vi "Math-updater-w--for-same-SpVar-names-03022016.vi"(0 "Sp_Id_Arr":string[](array[string]), 1 "Math Expressions":string[](array[string]), 2 "Pr_Id_Arr":string[](array[string]), 3 "LP-Cnt_4_Reac":string[](array[string]), 4 "LP_IDs":string[](array[string])) -> (5 "New Total Pr IDs":string[](array[string]), 6 "Math-w/-ch-VarID":string[](array[string]))   [LabVIEW 2014]
doc: "This VI checks if the variable and species name are same. If they are, then the math is updated with the new variable name in order to distinguish their value."
panel:
  out "j":i32
  out "k":i32
  out "New Pr IDs":string[](array[string])
  out "New LP IDs":string[](array[string])
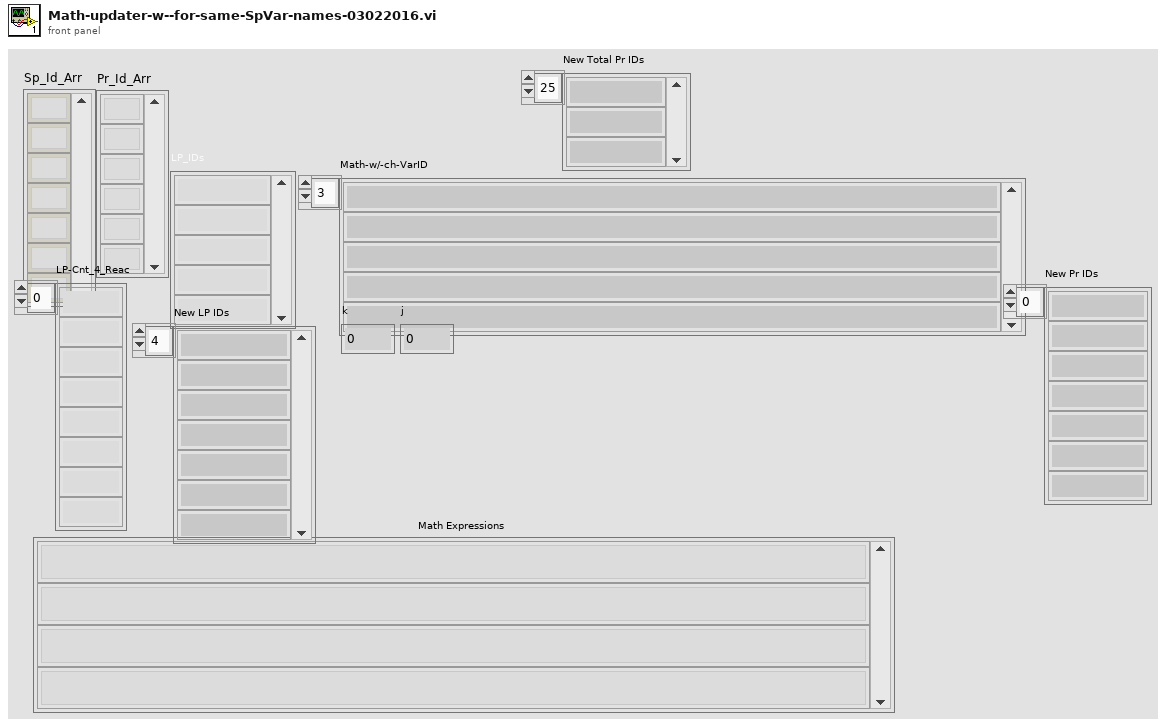
[diagram p1: front panel]
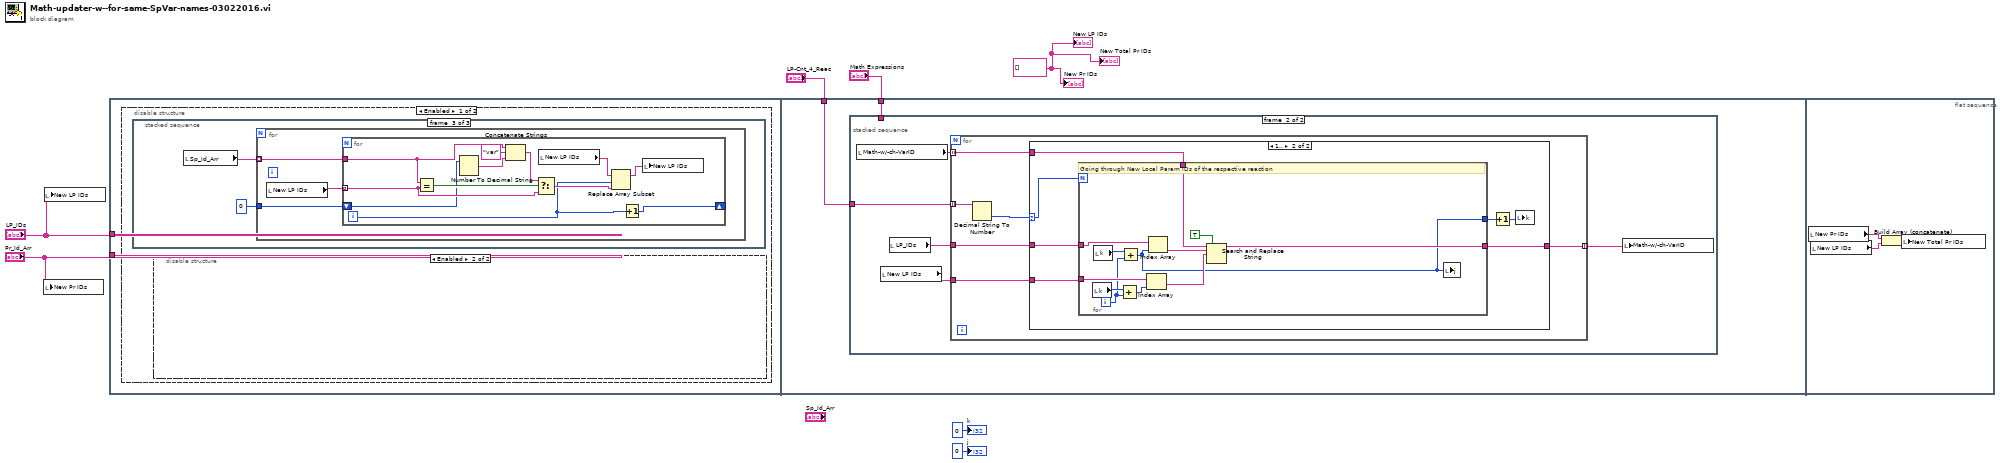
[diagram p0: block diagram]
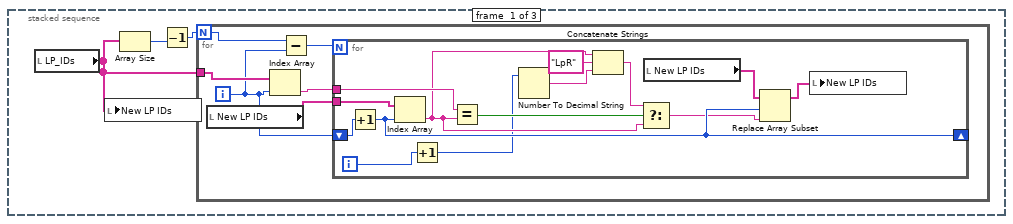
[diagram p2: hidden frame]
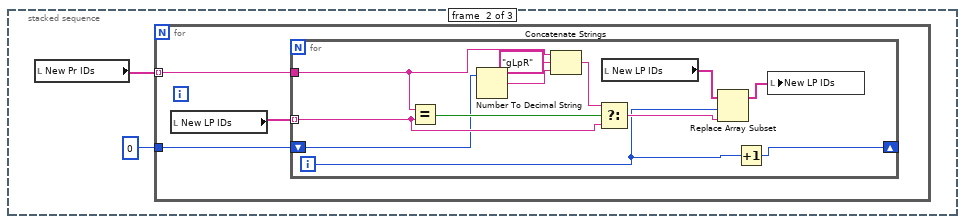
[diagram p3: hidden frame]
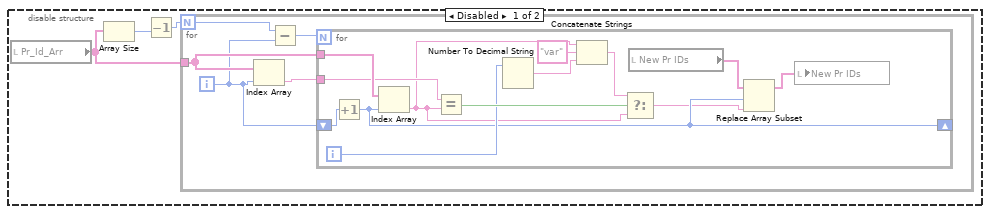
[diagram p4: hidden frame]
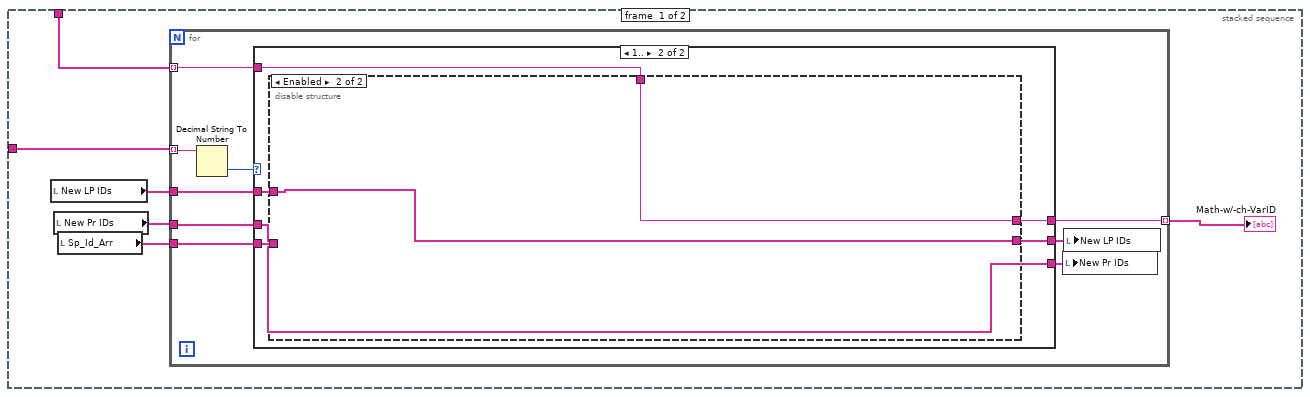
[diagram p6: hidden frame]
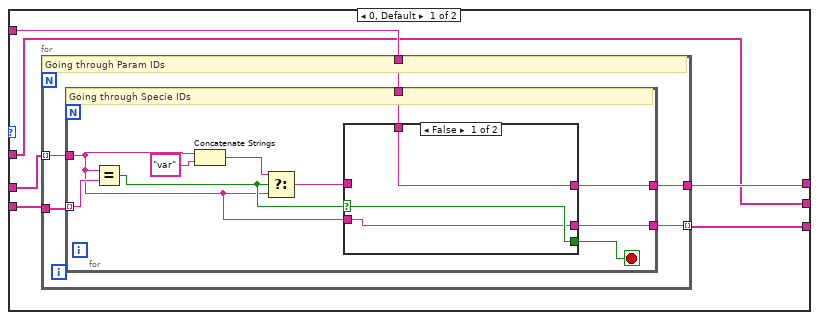
[diagram p7: hidden frame]
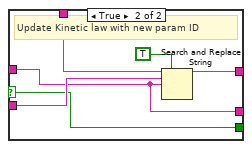
[diagram p8: hidden frame]
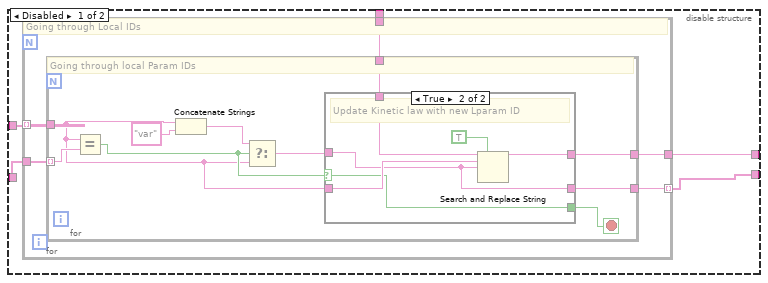
[diagram p9: hidden frame]
diagram:
  w7 = string[] [] ("New LP IDs")
  n1 = local write "New Pr IDs"("Pr_Id_Arr") -> ()
  n2 = local write "New LP IDs"("LP_IDs") -> ()
  n3 = flat-sequence {
    tunnel: "Pr_Id_Arr" -> [_]
    tunnel: "LP_IDs" -> [_]
    tunnel: "Math Expressions" -> [w87]
    tunnel: "LP-Cnt_4_Reac" -> [w86]
    frame #0 {
      n4 = disable-structure shown="Enabled" {
        frame Enabled {
          n5 = stacked-sequence {
            frame #0 {
              n6 = local read "LP_IDs"() -> (w8:string[])
              n7 = local write "New LP IDs"(w8) -> ()
              n8 = Array Size(array=w8) -> (size(s)=w10:i32)
              n9 = Decrement(x=w10) -> (x-1=w9:i32)
              n10 = for {
                N: w9 -> [w16]
                tunnel: w8 -> [w14]
                i -> [w12]
                n11 = local read "New LP IDs"() -> (w11:string[])
                n12 = Index Array(array=w14, index=w12) -> (element=w13:string)
                n13 = Subtract(x=w16, y=w12) -> (x-y=w15:i32)
                n14 = for {
                  N: w15 -> [_]
                  tunnel: w13 -> [w30]
                  shift-right: [w22] -> _
                  shift-left: w12 -> [w28]
                  tunnel: w11 -> [w17]
                  i -> [w19]
                  n15 = Increment(x=w28) -> (x+1=w22:i32)
                  n16 = Index Array(array=w17, index=w22) -> (element=w24:string)
                  n17 = Increment(x=w19) -> (x+1=w18:i32)
                  n18 = Equal?(x=w30, y=w24) -> (x = y?=w29:bool)
                  n19 = Number To Decimal String(number=w18) -> (decimal integer string=w25:string)  [unwired: 1 in]
                  n20 = Concatenate Strings(w24, "LpR" ("string"), w25) -> (w27:string)
                  n21 = Select(t=w27, s=w29, f=w24) -> (s? t:f=w21:string)
                  n22 = local read "New LP IDs"() -> (w23:string[])
                  n23 = Replace Array Subset(array=w23, new element=w21, index=w22) -> (w20:string[])
                  n24 = local write "New LP IDs"(w20) -> ()
                }
              }
            }
            frame #1 {
              n25 = local read "New Pr IDs"() -> (w32:string[])
              n26 = for {
                tunnel: w32 -> [w35] mode=indexing
                tunnel: 0 -> [w33]
                n27 = local read "New LP IDs"() -> (w34:string[])
                n28 = for {
                  tunnel: w35 -> [w40]
                  tunnel: w34 -> [w39] mode=indexing
                  shift-right: [w36] -> _
                  shift-left: w33 -> [w38]
                  i -> [w37]
                  n29 = Equal?(x=w40, y=w39) -> (x = y?=w47:bool)
                  n30 = Number To Decimal String(number=w38) -> (decimal integer string=w44:string)  [unwired: 1 in]
                  n31 = Concatenate Strings(w40, "gLpR" ("string"), w44) -> (w46:string)
                  n32 = Select(t=w46, s=w47, f=w39) -> (s? t:f=w42:string)
                  n33 = local read "New LP IDs"() -> (w43:string[])
                  n34 = Replace Array Subset(array=w43, new element=w42, index=w37) -> (w41:string[])
                  n35 = Increment(x=w37) -> (x+1=w36:i32)
                  n36 = local write "New LP IDs"(w41) -> ()
                }
              }
            }
            frame #2 {
              n37 = local read "Sp_Id_Arr"() -> (w49:string[])
              n38 = for {
                tunnel: w49 -> [w52] mode=indexing
                tunnel: 0 -> [w50]
                n39 = local read "New LP IDs"() -> (w51:string[])
                n40 = for {
                  tunnel: w52 -> [w57]
                  tunnel: w51 -> [w56] mode=indexing
                  shift-right: [w53] -> _
                  shift-left: w50 -> [w55]
                  i -> [w54]
                  n41 = Equal?(x=w57, y=w56) -> (x = y?=w64:bool)
                  n42 = Number To Decimal String(number=w55) -> (decimal integer string=w61:string)  [unwired: 1 in]
                  n43 = Concatenate Strings(w57, "var" ("string"), w61) -> (w63:string)
                  n44 = Select(t=w63, s=w64, f=w56) -> (s? t:f=w59:string)
                  n45 = local read "New LP IDs"() -> (w60:string[])
                  n46 = Replace Array Subset(array=w60, new element=w59, index=w54) -> (w58:string[])
                  n47 = Increment(x=w54) -> (x+1=w53:i32)
                  n48 = local write "New LP IDs"(w58) -> ()
                }
              }
            }
          }
          n49 = disable-structure shown="Enabled" {
            frame Disabled {
              n50 = local read "Pr_Id_Arr"() -> (w65:string[])
              n51 = Array Size(array=w65) -> (size(s)=w66:i32)
              n52 = Decrement(x=w66) -> (x-1=w67:i32)
              n53 = for {
                N: w67 -> [w72]
                tunnel: w65 -> [w70]
                i -> [w68]
                n54 = Index Array(array=w70, index=w68) -> (element=w69:string)
                n55 = Subtract(x=w72, y=w68) -> (x-y=w71:i32)
                n56 = for {
                  N: w71 -> [_]
                  tunnel: w70 -> [w85]
                  tunnel: w69 -> [w84]
                  shift-right: [w75] -> _
                  shift-left: w68 -> [w82]
                  i -> [w78]
                  n57 = Increment(x=w82) -> (x+1=w75:i32)
                  n58 = Index Array(array=w85, index=w75) -> (element=w77:string)
                  n59 = Equal?(x=w84, y=w77) -> (x = y?=w83:bool)
                  n60 = Number To Decimal String(number=w78) -> (decimal integer string=w79:string)  [unwired: 1 in]
                  n61 = Concatenate Strings(w77, "var" ("string"), w79) -> (w81:string)
                  n62 = Select(t=w81, s=w83, f=w77) -> (s? t:f=w74:string)
                  n63 = local read "New Pr IDs"() -> (w76:string[])
                  n64 = Replace Array Subset(array=w76, new element=w74, index=w75) -> (w73:string[])
                  n65 = local write "New Pr IDs"(w73) -> ()
                }
              }
            }
            frame Enabled {
            }
          }
        }
        frame Disabled {
        }
      }
    }
    frame #1 {
      n66 = stacked-sequence {
        tunnel: w87 -> [w93 _]
        tunnel: w86 -> [w92 w174]
        frame #0 {
          n67 = local read "New LP IDs"() -> (w91:string[])
          n68 = local read "New Pr IDs"() -> (w90:string[])
          n69 = local read "Sp_Id_Arr"() -> (w89:string[])
          n70 = for {
            tunnel: w93 -> [w98] mode=indexing
            tunnel: w92 -> [w102] mode=indexing
            tunnel: w91 -> [w100]
            tunnel: w89 -> [w99]
            tunnel: [w97] -> w88 mode=indexing
            tunnel: w90 -> [w96]
            n71 = Decimal String To Number(string=w102) -> (number=w101:i32)  [unwired: 2 in, 1 out]
            n72 = case shown="1.." w101 {
              tunnel: w100 -> [w103 w138]
              tunnel: w99 -> [w106 w137]
              tunnel: w98 -> [w107 w136]
              tunnel: [w108 w135] -> w97
              tunnel: w96 -> [w105 w134]
              tunnel: [w104 w134] -> w95
              tunnel: [w103 w133] -> w94
              frame 0, Default {
                n73 = for {
                  tunnel: w105 -> [w113] mode=indexing
                  tunnel: w106 -> [w112]
                  tunnel: w107 -> [w111]
                  tunnel: [w110] -> w108
                  tunnel: [w109] -> w104 mode=indexing
                  # "Going through Param IDs"
                  n74 = for {
                    tunnel: w113 -> [w117]
                    tunnel: w112 -> [w123] mode=indexing
                    tunnel: w111 -> [w118]
                    tunnel: [w116] -> w110
                    tunnel: [w114] -> w109
                    stop <- w115 stop-if-true
                    # "Going through Specie IDs"
                    n75 = Equal?(x=w117, y=w123) -> (x = y?=w120:bool)
                    n76 = Concatenate Strings(w117, "var") -> (w122:string)
                    n77 = Select(t=w122, s=w120, f=w117) -> (s? t:f=w119:string)
                    n78 = case shown="False" w120 {
                      selector: w120 -> [w125 w128]
                      tunnel: w119 -> [_ w127]
                      tunnel: w118 -> [w126 w131]
                      tunnel: w117 -> [w124 w130]
                      tunnel: [w126 w129] -> w116
                      tunnel: [w125 w128] -> w115
                      tunnel: [w124 w127] -> w114
                      frame False {
                      }
                      frame True {
                        # "Update Kinetic law with new param ID"
                        n79 = Search and Replace String(replace all?=TRUE ("replace all? (F)"), input string=w131, search string=w130, replace string=w127) -> (result string=w129:string)  [unwired: 4 in, 3 out]
                      }
                    }
                  }
                }
              }
              frame 1.. {
                n80 = disable-structure shown="Enabled" {
                  disable-tunnel: w138 -> [w143 w168]
                  disable-tunnel: w137 -> [w142 _]
                  disable-tunnel: w136 -> [w141 w169]
                  disable-tunnel: [w140 w169] -> w135
                  disable-tunnel: [w139 w168] -> w133
                  frame Disabled {
                    n81 = for {
                      tunnel: w143 -> [w148] mode=indexing
                      tunnel: w142 -> [w147]
                      tunnel: w141 -> [w146]
                      tunnel: [w145] -> w140
                      tunnel: [w144] -> w139 mode=indexing
                      # "Going through Local IDs"
                      n82 = for {
                        tunnel: w148 -> [w152]
                        tunnel: w147 -> [w158] mode=indexing
                        tunnel: w146 -> [w153]
                        tunnel: [w151] -> w145
                        tunnel: [w149] -> w144
                        stop <- w150 stop-if-true
                        # "Going through local Param IDs"
                        n83 = Equal?(x=w152, y=w158) -> (x = y?=w155:bool)
                        n84 = Concatenate Strings(w152, "var") -> (w157:string)
                        n85 = Select(t=w157, s=w155, f=w152) -> (s? t:f=w154:string)
                        n86 = case shown="True" w155 {
                          selector: w155 -> [w160 w163]
                          tunnel: w154 -> [_ w162]
                          tunnel: w153 -> [w161 w166]
                          tunnel: w152 -> [w159 w165]
                          tunnel: [w161 w164] -> w151
                          tunnel: [w160 w163] -> w150
                          tunnel: [w159 w162] -> w149
                          frame False {
                          }
                          frame True {
                            # "Update Kinetic law with new Lparam ID"
                            n87 = Search and Replace String(replace all?=TRUE ("replace all? (F)"), input string=w166, search string=w165, replace string=w162) -> (result string=w164:string)  [unwired: 4 in, 3 out]
                          }
                        }
                      }
                    }
                  }
                  frame Enabled {
                  }
                }
              }
            }
            n88 = local write "New Pr IDs"(w95) -> ()
            n89 = local write "New LP IDs"(w94) -> ()
          }
          "Math-w/-ch-VarID" <- w88
        }
        frame #1 {
          n90 = local read "Math-w/-ch-VarID"() -> (w171:string[])
          n91 = local read "New LP IDs"() -> (w172:string[])
          n92 = local read "LP_IDs"() -> (w170:string[])
          n93 = for {
            tunnel: w171 -> [w177] mode=indexing
            tunnel: w174 -> [w180] mode=indexing
            tunnel: w172 -> [w178]
            tunnel: [w176] -> w173 mode=indexing
            tunnel: w170 -> [w175]
            n94 = Decimal String To Number(string=w180) -> (number=w179:i32)  [unwired: 2 in, 1 out]
            n95 = case shown="1.." w179 {
              selector: w179 -> [_ w184]
              tunnel: w178 -> [_ w188]
              tunnel: w177 -> [w181 w187]
              tunnel: [w181 w186] -> w176
              tunnel: w175 -> [_ w185]
              frame 0, Default {
              }
              frame 1.. {
                n96 = for {
                  N: w184 -> [_]
                  tunnel: w188 -> [w197]
                  tunnel: w187 -> [w200]
                  tunnel: [w199] -> w186
                  tunnel: w185 -> [w193]
                  tunnel: [w189] -> w183
                  i -> [w192]
                  # "Going through New Local Param IDs of the respective reaction"
                  n97 = local read "k"() -> (w196:i32)
                  n98 = local read "k"() -> (w194:i32)
                  n99 = Add(x=w196, y=w192) -> (x+y=w195:i32)
                  n100 = Add(x=w194, y=w192) -> (x+y=w189:i32)
                  n101 = Index Array(array=w197, index=w195) -> (element=w190:string)
                  n102 = Index Array(array=w193, index=w189) -> (element=w191:string)
                  n103 = Search and Replace String(replace all?=TRUE ("replace all? (F)"), input string=w200, search string=w191, replace string=w190) -> (result string=w199:string)  [unwired: 4 in, 3 out]
                  n104 = local write "j"(w189) -> ()
                }
                n105 = Increment(x=w183) -> (x+1=w182:i32)
                n106 = local write "k"(w182) -> ()
              }
            }
          }
          n107 = local write "Math-w/-ch-VarID"(w173) -> ()
        }
      }
    }
    frame #2 {
      n108 = local read "New Pr IDs"() -> (w202:string[])
      n109 = local read "New LP IDs"() -> (w203:string[])
      n110 = Build Array (concatenate)(w202, w203) -> (w201:string[])
      n111 = local write "New Total Pr IDs"(w201) -> ()
    }
  }
  "New LP IDs" <- w7
  "New Pr IDs" <- w7
  "New Total Pr IDs" <- w7
  "k" <- 0 ("LP Off")
  "j" <- 0 ("LP Off")
